vi "Pic to XY (SubVI).vi"(11 "Picture":i32[][](array[numeric])) -> (2 "Y distance":i32(slide) scale=0.0..100.0, 3 "X distance":i32(slide) scale=0.0..100.0)   [LabVIEW 2013]
doc: "Derive the X, Y distance between the bird and the gap from the picture."
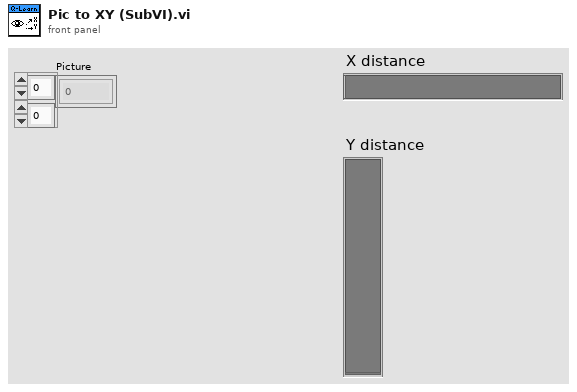
[diagram p1: front panel]
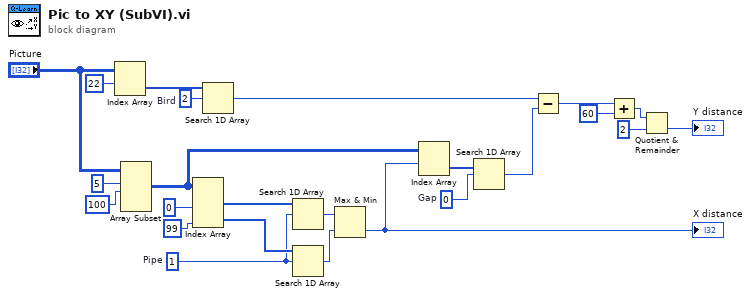
[diagram p0: block diagram]
diagram:
  w7 = 0  # Gap
  w11 = 1  # Pipe
  w23 = 2  # Bird
  n1 = Index Array(array="Picture", index (row)=22 ("disabled index (col)")) -> (element=w24:i32[])  [unwired: 1 in]
  n2 = Array Subset(array="Picture", index (row)=5 ("index"), length (row)=100 ("length")) -> (w10:i32[][])  [unwired: 2 in]
  n3 = Index Array(array=w10, index (col) #1=0 ("disabled index (col)"), index (col) #2=99 ("index (col)")) -> (element #1=w16:i32[], element #2=w15:i32[])  [unwired: 2 in]
  n4 = Search 1D Array(1D array=w24, element=w23) -> (index of element=w22:i32)  [unwired: 1 in]
  n5 = Search 1D Array(1D array=w16, element=w11) -> (index of element=w14:i32)  [unwired: 1 in]
  n6 = Search 1D Array(1D array=w15, element=w11) -> (index of element=w13:i32)  [unwired: 1 in]
  n7 = Max & Min(x=w14, y=w13) -> (min(x,y)=w9:i32)  [unwired: 1 out]
  "X distance" <- w9
  n8 = Index Array(array=w10, index (row)=w9) -> (element=w8:i32[])  [unwired: 1 in]
  n9 = Search 1D Array(1D array=w8, element=w7) -> (index of element=w6:i32)  [unwired: 1 in]
  n10 = Subtract(x=w22, y=w6) -> (x-y=w2:i32)
  n11 = Add(x=w2, y=60) -> (x+y=w4:i32)
  n12 = Quotient & Remainder(x=w4, y=2) -> (floor(x/y)=→"Y distance":i32)  [unwired: 1 out]
